vi "Run Application.vi"(3 "working directory":path, 6 "timeout (ms) (60000)":i32=60000, 8 "error in (no error)":errorcluster, 9 "wait until closed? (F)":bool, 10 "run minimized? (F)":bool, 11 "command line to execute (\"\")":string) -> (0 "error out":errorcluster, 2 "window names":string[](array[string]))   [LabVIEW 2023, in "Winevent.lvlib"]
doc: "This VI will launch another application as if you used the Run... command from Program Manager's or File Manager's File menu. If the wait until closed? setting is TRUE, the VI will wait until you close the application before continuing. The names of Task List windows are returned in the window names array.\n\nYou can also choose how the window for the application will appear (for Windows applications only) with the run minimized? input.\n\nIf an error occurs, the code is returned in the error cluster."
uses:
  Winevent.lvlib
  LVWUtil32.dll
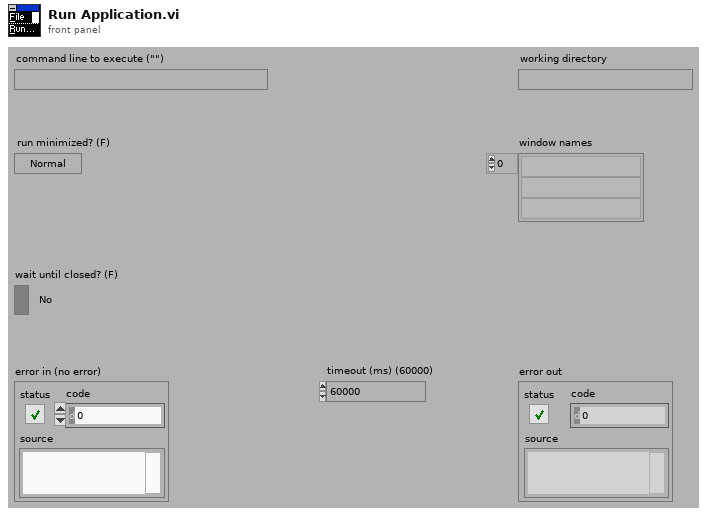
[diagram p1: front panel]
types:
  T1 = enum16{"Get Number of Tasks", "Get Window Info", "Get Window Names"}
  T2 = cluster{"number of windows":i32, "total names length":u32, "number of tasks found":i32, "window handles":u32[], "process ID":u32}
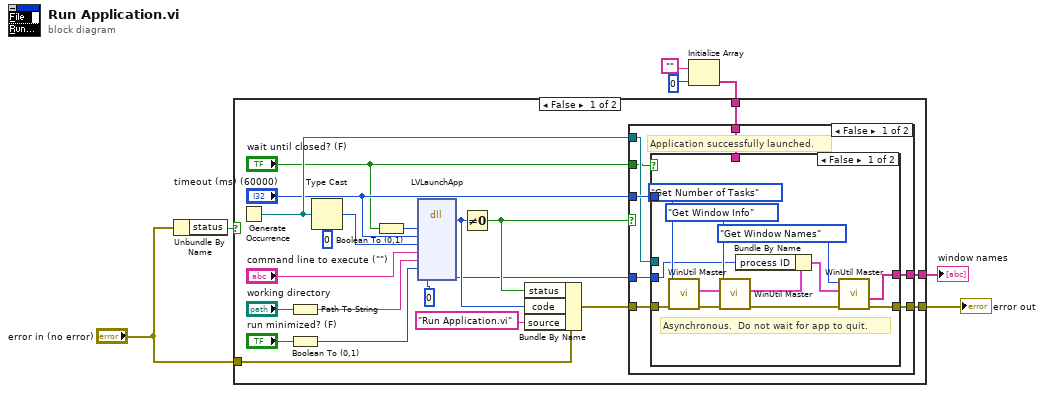
[diagram p0: block diagram]
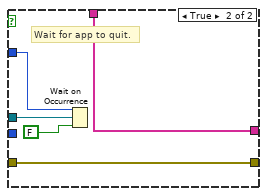
[diagram p2: hidden frame]
diagram:
  n1 = Unbundle By Name("error in (no error)") -> ("status"=w7:bool)
  n2 = Initialize Array("", 0) -> (w4:string[])
  n3 = case shown="False" w7 {
    tunnel: "error in (no error)" -> [w27 w59]
    tunnel: [w24 w59] -> w1
    tunnel: [w23 w57] -> w6
    tunnel: w4 -> [w8 _]
    frame False {
      n4 = Generate Occurrence() -> (w12:refnum<k4>)
      n5 = Path To String(path="working directory") -> (string=w15:string)
      n6 = Boolean To (0,1)(Boolean="run minimized? (F)") -> (0, 1=w14:i16)
      n7 = Type Cast(type=0, x=w12) -> (*(type *) &x=w18:i32)
      n8 = Boolean To (0,1)(Boolean="wait until closed? (F)") -> (0, 1=w20:i16)
      n9 = dll-call lib="C:/Users/acasalen/Documents/LabVIEW Data/Projects/Reds-Auto-Clicker/Red's Auto Clicker/SubVIs/labview_win_util32_8.6/LVWUtil32.dll" fn="LVLaunchApp"("bWait"=w20, "lTimeout"="timeout (ms) (60000)", "oRefNum"=w18, "lpszCommandLine"="command line to execute (\"\")", "lpszWorkDir"=w15, "bRunMinimized"=w14, "processId"=u32 0) -> (w21:i32, "processId"=w9:u32)  [unwired: 9 in, 2 out]
      n10 = Not Equal To 0?(x=w21) -> (x != 0?=w22:bool)
      n11 = Bundle By Name(cluster=w27, "status"=w22, "code"=w21, "source"="Run Application.vi") -> (w25:errorcluster)
      n12 = case shown="False" w22 {
        tunnel: w25 -> [w36 w55]
        tunnel: [w35 w55] -> w24
        tunnel: [w34 w54] -> w23
        tunnel: w12 -> [w32 _]
        tunnel: "timeout (ms) (60000)" -> [w33 _]
        tunnel: "wait until closed? (F)" -> [w31 _]
        tunnel: w9 -> [w30 _]
        tunnel: w8 -> [w29 w54]
        frame False {
          # "Application successfully launched."
          n13 = case shown="False" w31 {
            tunnel: w36 -> [w46 w53]
            tunnel: [w45 w53] -> w35
            tunnel: [w40 w49] -> w34
            tunnel: w33 -> [_ w50]
            tunnel: w32 -> [_ w51]
            tunnel: w30 -> [w37 _]
            tunnel: w29 -> [_ w49]
            frame False {
              # "Asynchronous.  Do not wait for app to quit."
              n14 = call "WinUtil Master.vi"("error in (no error)"=w46, "function"=T1."Get Number of Tasks") -> ("error out"=w48:errorcluster, "window enumeration info out"=w44:T2)  [unwired: 7 in, 1 out]
              n15 = call "WinUtil Master.vi"("error in (no error)"=w48, "window enumeration info in"=w44, "function"=T1."Get Window Info") -> ("error out"=w47:errorcluster, "window enumeration info out"=w41:T2)  [unwired: 6 in, 1 out]
              n16 = Bundle By Name(cluster=w41, "process ID"=w37) -> (w39:T2)
              n17 = call "WinUtil Master.vi"("error in (no error)"=w47, "window enumeration info in"=w39, "function"=T1."Get Window Names") -> ("error out"=w45:errorcluster, "window names"=w40:string[])  [unwired: 6 in, 1 out]
            }
            frame True {
              # "Wait for app to quit."
              n18 = Wait on Occurrence(1:FALSE, 2:w51, 3:w50) -> ()  [unwired: 1 out]
            }
          }
        }
        frame True {
          # "Error"
        }
      }
    }
    frame True {
      # "Error in.  Do nothing."
      n19 = Initialize Array("", 0) -> (w57:string[])
    }
  }
  "window names" <- w6
  "error out" <- w1
